vi "itc Hg box controller -- wrapper -- A1.vi"(6 "Log File Path":path, 7 "itc box action":T3=enum."init", 8 "error in":errorcluster, 9 "Sweep Table In":dbl[][](array[numeric])=[[650.0, 1334.0, 30.0], [300.0, 1334.0, 0.0], [0.0, 0.0, 0.0], [0.0, 0.0, 0.0], [0.0, 0.0, 0.0], [0.0, 0.0, 0.0], [0.0, 0.0, 0.0], [0.0, 0.0, 0.0], [0.0, 0.0, 0.0], [0.0, 0.0, 0.0], [0.0, 0.0, 0.0], [300.0, 0.0, 0.0], [0.0, 0.0, 0.0], [0.0, 0.0, 0.0], [0.0, 0.0, 0.0], [300.0, 0.0, 0.0]], 10 "input":dbl=10.0, 11 "VISA resource name":refnum<visa-resource-name>="GPIB0::1::INSTR") -> (0 "error out":errorcluster, 1 "Sweep Table":dbl[][](array[numeric])=[[650.0, 1334.0, 30.0], [300.0, 1334.0, 0.0], [0.0, 0.0, 0.0], [0.0, 0.0, 0.0], [0.0, 0.0, 0.0], [0.0, 0.0, 0.0], [0.0, 0.0, 0.0], [0.0, 0.0, 0.0], [0.0, 0.0, 0.0], [0.0, 0.0, 0.0], [0.0, 0.0, 0.0], [300.0, 0.0, 0.0], [0.0, 0.0, 0.0], [0.0, 0.0, 0.0], [0.0, 0.0, 0.0], [300.0, 0.0, 0.0]], 2 "itc box state OUT":T2={"ITC503 Address"="GPIB0::15::INSTR", "ITC temperature"=0.0, "ITC set temperature"=300.0, "heater"=300.0, "gas flow"=1.6, "P"=0.0, "D"=10.0, "I"=0.1, "ITC state"="X0A1C2S01H1L0\r", "nonzero temperature"=0.0, "Magn Field (T)"=0.0})   [LabVIEW 2015]
uses:
  itc 503 box - control.ctl
  itc 503 box state.ctl
  oxford ITC legacy-new - control.ctl
  mercury ixx/public/Controls/ISOBus Address.ctl
  mercury ixx/Mercury iXX.lvlib
panel:
  out "Tab Control":T1(tab)
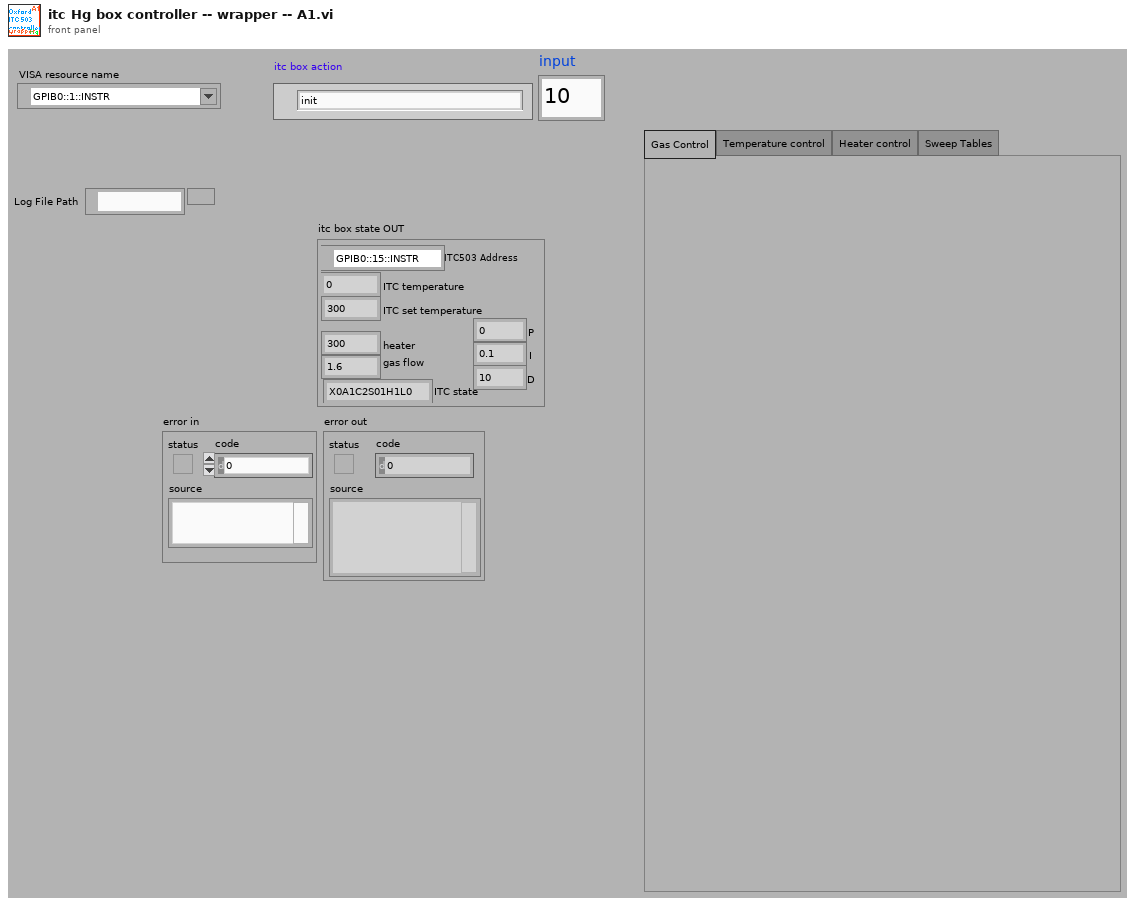
[diagram p1: front panel]
types:
  T1 = enum32{"Gas Control", "Temperature control", "Heater control", "Sweep Tables"}
  T2 = typedef "itc 503 box state.ctl" = cluster{"ITC503 Address":refnum<visa-resource-name>, "ITC temperature":dbl, "ITC set temperature":dbl, "heater":dbl, "gas flow":dbl, "P":dbl, "D":dbl, "I":dbl, "ITC state":string, "nonzero temperature":dbl, "Magn Field (T)":dbl}
  T3 = typedef "itc 503 box - control.ctl" = enum16{"heater manual and zero", "heater auto", "upload D", "upload I", "upload P", "shut off", "init", "read sweep table", "disable", "enable", "read state", "set gas to", "stop sweep", "start sweep", "test", "set temperature to", "write sweep table", "-void", "set heater to"}
  T4 = typedef "oxford ITC legacy-new - control.ctl" = enum16{"legacy", "new"}
  T5 = typedef "Mercury iXX.lvlib/ISOBus Address.ctl" = i32
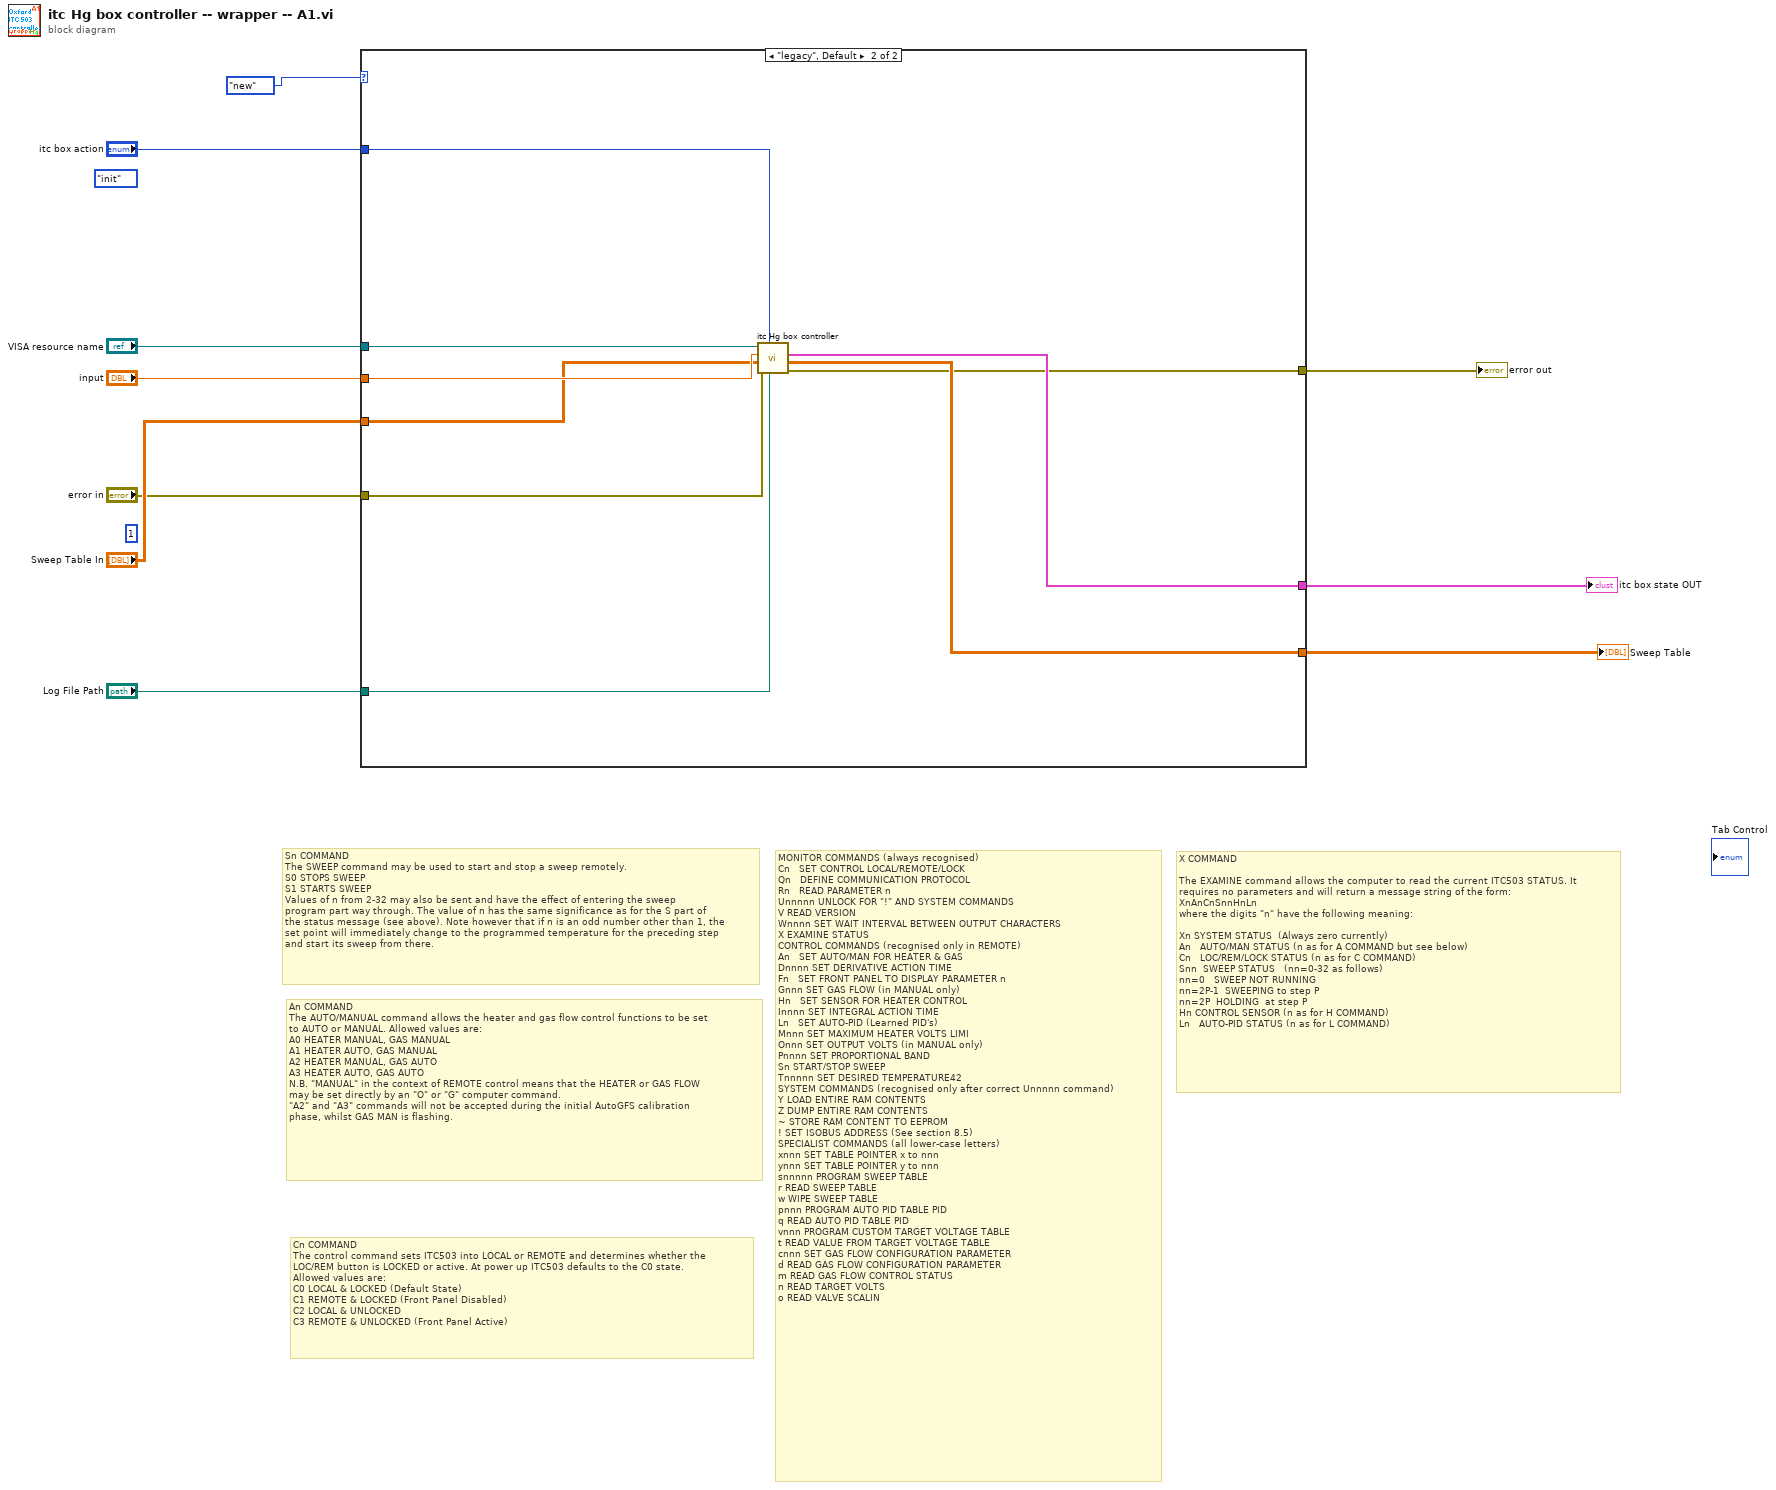
[diagram p0: block diagram]
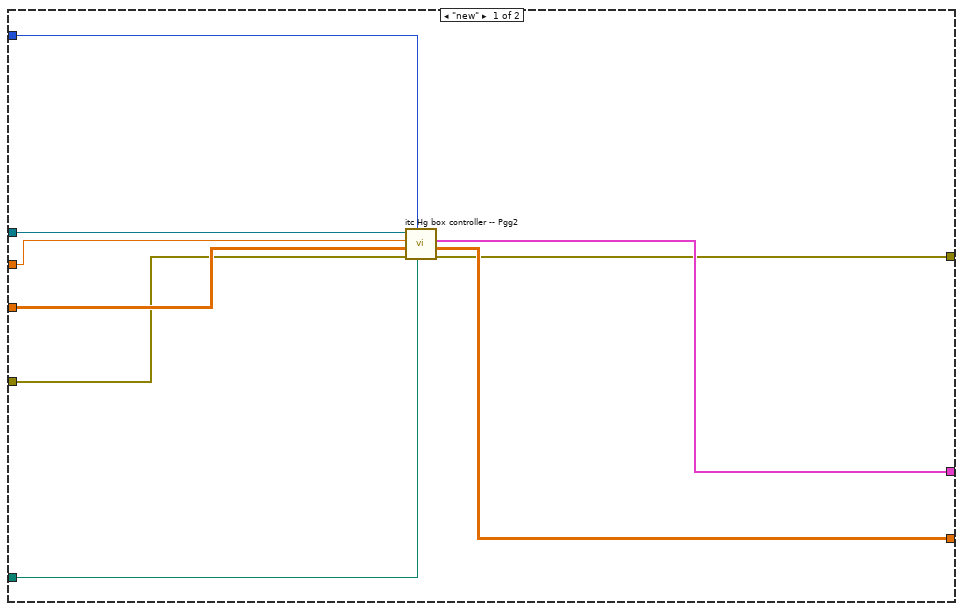
[diagram p2: hidden frame]
diagram:
  (unwired) T5 1 ("ISOBUS address")
  (unwired) itc_503_box_-_control."init" ("itc box action")
  # "Cn COMMAND\nThe control command sets ITC503 into LOCAL or REMOTE and determines whether the\nLOC/REM button is LOCKED or active. At power up ITC503 defaults to the C0 state.\nAllowed values are:\nC0 LOCAL & LOCKED (Default State)\nC1 REMOTE & LOCKED (Front Panel Disabled)\nC2 LOCAL & UNLOCKED\nC3 REMOTE & UNLOCKED (Front Panel Active)"
  # "An COMMAND\nThe AUTO/MANUAL command allows the heater and gas flow control functions to be set\nto AUTO or MANUAL. Allowed values are:\nA0 HEATER MANUAL, GAS MANUAL\nA1 HEATER AUTO, GAS MANUAL\nA2 HEATER MANUAL, GAS AUTO\nA3 HEATER AUTO, GAS AUTO\nN.B. \"MANUAL\" in the context of REMOTE control means that the HEATER or GAS FLOW\nmay be set directly by an \"O\" or \"G\" computer command.\n\"A2\" and \"A3\" commands will not be accepted during the initial AutoGFS calibration\nphase, whilst GAS MAN is flashing."
  # "MONITOR COMMANDS (always recognised)\nCn   SET CONTROL LOCAL/REMOTE/LOCK\nQn   DEFINE COMMUNICATION PROTOCOL\nRn   READ PARAMETER n\nUnnnnn UNLOCK FOR \"!\" AND SYSTEM COMMANDS\nV READ VERSION\nWnnnn SET WAIT INTERVAL BETWEEN OUTPUT CHARACTERS\nX EXAMINE STATUS\nCONTROL COMMANDS (recognised only in REMOTE)\nAn   SET AUTO/MAN FOR HEATER & GAS\nDnnnn SET DERIVATIVE ACTION TIME\nFn   SET FRONT PANEL TO DISPLAY PARAMETER n\nGnnn SET GAS FLOW (in MANUAL only)\nHn   SET SENSOR FOR HEATER CONTROL\nInnnn SET INTEGRAL ACTION TIME\nLn   SET AUTO-PID (Learned PID's)\nMnnn SET MAXIMUM HEATER VOLTS LIMI\nOnnn SET OUTPUT VOLTS (in MANUAL only)\nPnnnn SET PROPORTIONAL BAND\nSn START/STOP SWEEP\nTnnnnn SET DESIRED TEMPERATURE42\nSYSTEM COMMANDS (recognised only after correct Unnnnn command)\nY LOAD ENTIRE RAM CONTENTS\nZ DUMP ENTIRE RAM CONTENTS\n~ STORE RAM CONTENT TO EEPROM\n! SET ISOBUS ADDRESS (See section 8.5)\nSPECIALIST COMMANDS (all lower-case letters)\nxnnn SET TABLE POINTER x to nnn\nynnn SET TABLE POINTER y to nnn\nsnnnnn PROGRAM SWEEP TABLE\nr READ SWEEP TABLE\nw WIPE SWEEP TABLE\npnnn PROGRAM AUTO PID TABLE PID\nq READ AUTO PID TABLE PID\nvnnn PROGRAM CUSTOM TARGET VOLTAGE TABLE\nt READ VALUE FROM TARGET VOLTAGE TABLE\ncnnn SET GAS FLOW CONFIGURATION PARAMETER\nd READ GAS FLOW CONFIGURATION PARAMETER\nm READ GAS FLOW CONTROL STATUS\nn READ TARGET VOLTS\no READ VALVE SCALIN"
  # "X COMMAND\n\nThe EXAMINE command allows the computer to read the current ITC503 STATUS. It\nrequires no parameters and will return a message string of the form:\nXnAnCnSnnHnLn\nwhere the digits \"n\" have the following meaning:\n\nXn SYSTEM STATUS  (Always zero currently)\nAn   AUTO/MAN STATUS (n as for A COMMAND but see below)\nCn   LOC/REM/LOCK STATUS (n as for C COMMAND)\nSnn  SWEEP STATUS   (nn=0-32 as follows)\nnn=0   SWEEP NOT RUNNING\nnn=2P-1  SWEEPING to step P\nnn=2P  HOLDING  at step P\nHn CONTROL SENSOR (n as for H COMMAND)\nLn   AUTO-PID STATUS (n as for L COMMAND)"
  # "Sn COMMAND\nThe SWEEP command may be used to start and stop a sweep remotely.\nS0 STOPS SWEEP\nS1 STARTS SWEEP\nValues of n from 2-32 may also be sent and have the effect of entering the sweep\nprogram part way through. The value of n has the same significance as for the S part of\nthe status message (see above). Note however that if n is an odd number other than 1, the\nset point will immediately change to the programmed temperature for the preceding step\nand start its sweep from there."
  n1 = case shown="\"legacy\", Default" oxford_ITC_legacy-new_-_control."new" ("itc box protocol selector") {
    tunnel: "itc box action" -> [w19 w28]
    tunnel: "VISA resource name" -> [w18 w27]
    tunnel: "input" -> [w17 w26]
    tunnel: "Sweep Table In" -> [w16 w25]
    tunnel: "error in" -> [w15 w24]
    tunnel: "Log File Path" -> [w14 w23]
    tunnel: [w13 w22] -> w3
    tunnel: [w12 w21] -> w2
    tunnel: [w11 w20] -> w1
    frame "new" {
      n2 = call "itc Hg box controller -- Pgg2.vi"("Log File Path"=w14, "itc box action"=w19, "error in"=w15, "Sweep Table In"=w16, "input"=w17, "VISA resource name"=w18) -> ("error out"=w11:errorcluster, "Sweep Table"=w12:dbl[][], "itc box state OUT"=w13:T2)  [unwired: 3 in]
    }
    frame "legacy", Default {
      n3 = call "itc Hg box controller.vi"("Log File Path"=w23, "itc box action"=w28, "error in"=w24, "Sweep Table In"=w25, "input"=w26, "VISA resource name"=w27) -> ("error out"=w20:errorcluster, "Sweep Table"=w21:dbl[][], "itc box state OUT"=w22:T2)  [unwired: 3 in]
    }
  }
  "itc box state OUT" <- w3
  "Sweep Table" <- w2
  "error out" <- w1
